vi "BuildPlotLegends.vi"(9 "Plot selecter \n    1      2     3     4":bool[][](array[boolean])=[[FALSE, TRUE, FALSE, FALSE], [FALSE, FALSE, FALSE, FALSE], [FALSE, FALSE, FALSE, FALSE], [FALSE, FALSE, FALSE, TRUE], [TRUE, FALSE, FALSE, FALSE], [FALSE, FALSE, FALSE, FALSE], [FALSE, FALSE, FALSE, FALSE], [FALSE, TRUE, FALSE, FALSE], [FALSE, TRUE, FALSE, FALSE], [FALSE, TRUE, FALSE, FALSE], [FALSE, TRUE, FALSE, FALSE], [FALSE, FALSE, FALSE, FALSE], [FALSE, FALSE, FALSE, FALSE], [FALSE, FALSE, FALSE, FALSE], [FALSE, FALSE, FALSE, FALSE], [FALSE, FALSE, FALSE, FALSE], [FALSE, FALSE, FALSE, FALSE], [FALSE, FALSE, FALSE, FALSE], [FALSE, FALSE, FALSE, FALSE], [FALSE, FALSE, FALSE, FALSE], [FALSE, FALSE, FALSE, FALSE], [FALSE, FALSE, FALSE, FALSE], [FALSE, FALSE, FALSE, FALSE], [FALSE, FALSE, FALSE, FALSE]], 11 "AllLabels":string[](array[string])=["GXS450", "Vacuum insluation", "LeakDet_EXP", "LeakDet_Mantissa", "LaekDet_FULL"]) -> (0 "Series 4":string[](array[string]), 1 "Series 3":string[](array[string]), 2 "Series 2":string[](array[string]), 3 "Series 1":string[](array[string]))   [LabVIEW 2017]
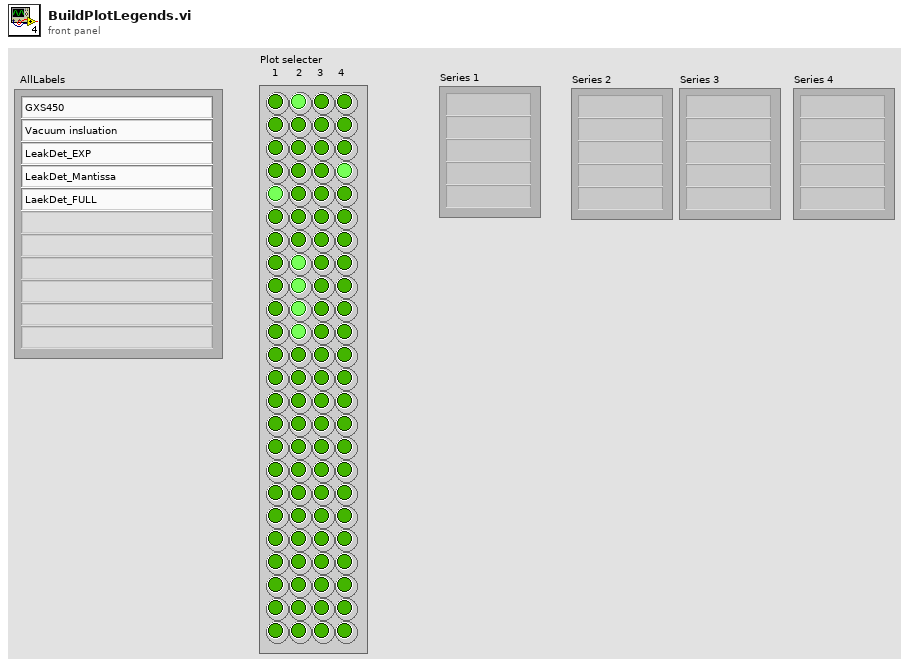
[diagram p1: front panel]
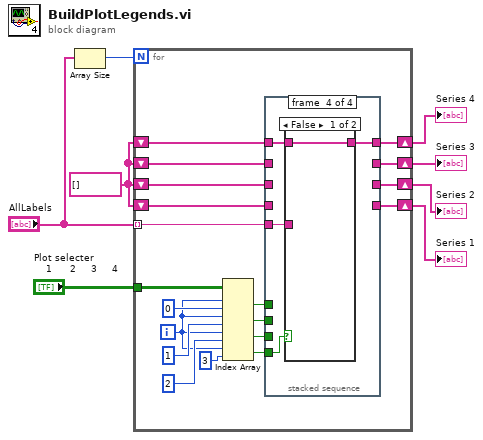
[diagram p0: block diagram]
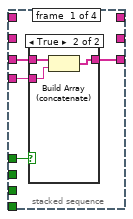
[diagram p2: hidden frame]
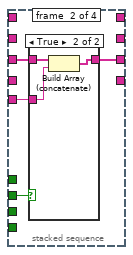
[diagram p4: hidden frame]
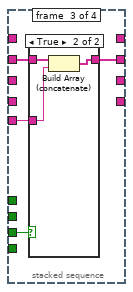
[diagram p6: hidden frame]
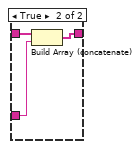
[diagram p8: hidden frame]
diagram:
  w6 = string[] []
  n1 = Array Size(array="AllLabels") -> (size(s)=w8:i32)
  n2 = for {
    N: w8 -> [_]
    shift-right: [w10] -> w4
    shift-left: w6 -> [w27]
    shift-right: [w12] -> w2
    shift-left: w6 -> [w26]
    shift-right: [w11] -> w3
    shift-left: w6 -> [w25]
    shift-right: [w9] -> w1
    shift-left: w6 -> [w24]
    tunnel: "Plot selecter \n    1      2     3     4" -> [w14]
    tunnel: "AllLabels" -> [w13] mode=indexing
    i -> [w19]
    n3 = Index Array(array=w14, index (row) #1=w19, index (col) #1=0 ("index (row)"), index (row) #2=w19, index (col) #2=1 ("index (row)"), index (row) #3=w19, index (col) #3=2 ("index (row)"), index (row) #4=w19, index (col) #4=3 ("index (row)")) -> (element #1=w18:bool, element #2=w17:bool, element #3=w16:bool, element #4=w15:bool)
    n4 = stacked-sequence {
      tunnel: w18 -> [w28 _ _ _]
      tunnel: [w31 _ _ _] -> w10
      tunnel: w16 -> [_ _ w44 _]
      tunnel: [_ _ w47 _] -> w12
      tunnel: w15 -> [_ _ _ w52]
      tunnel: [_ _ _ w55] -> w9
      tunnel: w27 -> [w30 _ _ _]
      tunnel: w26 -> [_ _ w46 _]
      tunnel: [_ w39 _ _] -> w11
      tunnel: w25 -> [_ w38 _ _]
      tunnel: w24 -> [_ _ _ w54]
      tunnel: w17 -> [_ w36 _ _]
      tunnel: w13 -> [w29 w37 w45 w53]
      frame #0 {
        n5 = case shown="True" w28 {
          tunnel: [w32 w35] -> w31
          tunnel: w30 -> [w32 w34]
          tunnel: w29 -> [_ w33]
          frame False {
          }
          frame True {
            n6 = Build Array (concatenate)(w34, w33) -> (w35:string[])
          }
        }
      }
      frame #1 {
        n7 = case shown="True" w36 {
          tunnel: [w40 w43] -> w39
          tunnel: w38 -> [w40 w42]
          tunnel: w37 -> [_ w41]
          frame False {
          }
          frame True {
            n8 = Build Array (concatenate)(w42, w41) -> (w43:string[])
          }
        }
      }
      frame #2 {
        n9 = case shown="True" w44 {
          tunnel: [w48 w51] -> w47
          tunnel: w46 -> [w48 w50]
          tunnel: w45 -> [_ w49]
          frame False {
          }
          frame True {
            n10 = Build Array (concatenate)(w50, w49) -> (w51:string[])
          }
        }
      }
      frame #3 {
        n11 = case shown="False" w52 {
          tunnel: [w56 w59] -> w55
          tunnel: w54 -> [w56 w58]
          tunnel: w53 -> [_ w57]
          frame False {
          }
          frame True {
            n12 = Build Array (concatenate)(w58, w57) -> (w59:string[])
          }
        }
      }
    }
  }
  "Series 1" <- w4
  "Series 2" <- w3
  "Series 3" <- w2
  "Series 4" <- w1
